vi "Test Host Image Acquisition Module Random Data No Accumulation.vi"(8 "error in":errorcluster, 11 "Operation":T3) -> (0 "error out":errorcluster, 1 "Image Acquired":bool, 2 "Acq In Progress":bool, 3 "Image":T2(plugin-control))   [LabVIEW 2013]
uses:
  Host/Image Acquisition/Host Image Acquisition Module Enum.ctl
  Host/Image Acquisition/Acquisition Settings Cluster.ctl
  <vilib>/vision/Image Controls.llb/IMAQ Image.ctl
  Host/Image Acquisition/Image Acquisition Settings FG Enum.ctl
  Host/System Status/Status FG Enum.ctl
  Host/Image Processing/Mask ROI FG Enum.ctl
  <vilib>/Utility/error.llb/Error Cluster From Error Code.vi
  <vilib>/rvi/errors/niLvFpgaAdjustHostInterfaceError.vi
  <vilib>/FPGAPlugInAG/PCIe-7842R/niLvFpga_Run_PCIe-7842R.vi
  <vilib>/FPGAPlugInAG/PCIe-7842R/niLvFpga_Close_PCIe-7842R.vi
  <vilib>/rvi/interface/nirviReadWriteControl/nirviReadWriteControl.xnode
  Host/FGs/FPGA_Reference.ctl
  Common/CL Configuration.ctl
  Common/CL Signal Mapping.ctl
  FPGA Bitfiles/WingBeatAnalyzer_FPGATargetSim_10_2.lvbitx
  <vilib>/rvi/interface/nirviMethod/nirviMethod.xnode
  FPGA/Sector/Accumulate/Sector Parameter Cluster.ctl
  <vilib>/rvi/interface/nirviCloseFPGA/nirviCloseFPGA.xnode
  Common/Timing/Timing Lib.lvlib
  Host/Globals/Average Sector Data.vi
  NiFpgaLv.dll
  <vilib>/FPGAPlugInAG/PCIe-7842R/niLvFpga_ConfigureFifo_PCIe-7842R.vi
  <vilib>/rvi/errors/niLvFpgaMergeErrorWithErrorCode.vi
  <vilib>/FPGAPlugInAG/PCIe-7842R/niLvFpga_StartFifo_PCIe-7842R.vi
  <vilib>/FPGAPlugInAG/PCIe-7842R/niLvFpga_ReadFifo_PCIe-7842R.vi
  <vilib>/FPGAPlugInAG/PCIe-7842R/niLvFpga_Reset_PCIe-7842R.vi
panel:
  out "Actual Depth":u32
  out "Target Sim TO":bool
  out "Cam Data Timeout":bool
  out "Sector FIFO Timeout":bool
  out "Host DMA Timeout":bool
  out "Number of Elements to Write Host DMA":u32
  out "Number of Elements to Read Cam Data":u32
  out "Image Data":u64[](array[numeric])
  out "Elements Remaining":u32
  out "Words per image":u32
  out "Num Frames read":u32
  out "DMA Words per Image":u32
  out "Acquire":bool
  in  "Acquisition Settings Cluster":T1={"Image Width"=2040, "Image Height"=1088, "Frames To Acquire"=0, "Signal Mapping"=enum."Basler 10-tap", "DMA Buffer Size\n(In Images)"=64} {"Image Height" max=65535; "Image Width" max=65535 step=40}
  out "Buffer Size":u32
  out "Acq'd Frame Width":u32=2040
  out "DMA Write Timeout":bool
  in  "Start Serial Server":bool
  out "Frames Acq'd":u32=1
  out "Acq'd Frame Height":u32=1088
  out "Initialized":bool
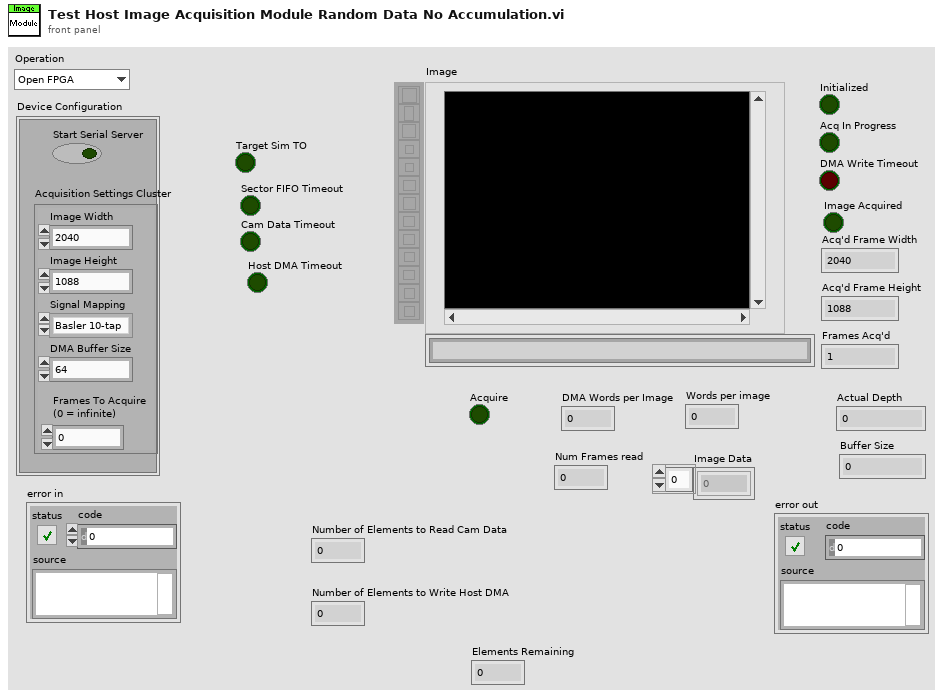
[diagram p1: front panel]
types:
  T1 = typedef "Acquisition Settings Cluster.ctl" = cluster{"Image Width":u32, "Image Height":u32, "Frames To Acquire":u32, "Signal Mapping":enum8{"Standard", "Basler 10-tap", "Vosskühler 10-tap"}, "DMA Buffer Size\n(In Images)":u32}
  T2 = typedef "IMAQ Image.ctl" = refnum<image>
  T3 = typedef "Host Image Acquisition Module Enum.ctl" = enum16{"Open FPGA", "Initialize DMA FIFO", "Load Sim Images", "Initialize Acquisition", "Update Sector Parameters", "Start Acquisition", "Aquire Image", "Read Averages", "Cancel Acquisition", "Close FPGA"}
  T4 = enum8{"Standard", "Basler 10-tap", "Vosskühler 10-tap"}
  T5 = typedef "Image Acquisition Settings FG Enum.ctl" = enum16{"Read", "Write"}
  T6 = typedef "Status FG Enum.ctl" = enum16{"Reset", "Read", "Write"}
  T7 = typedef "Mask ROI FG Enum.ctl" = enum16{"Read", "Write"}
  T8 = enum16{"big-endian, network order", "native, host order", "little-endian"}
  T9 = typedef "FPGA_Reference.ctl" = refnum<k20>
  T10 = typedef "Image Type" = u32
  T11 = typedef "Mask ROI Cluster.ctl" = cluster{"left annulus":T12, "right annulus":T12, "Threshold Range":cluster{"Lower value":dbl, "Upper value":dbl}, "[Avg BG]":u8[], "Number of Sectors":u8, "Left ROI":T13, "Right ROI":T13, "Left Start Angle Duty Cycle":fxp<+,8,0>, "Left End Angle Duty Cycle":fxp<+,8,0>, "Right End Angle Duty Cycle":fxp<+,8,0>, "Right Start Angle Duty Cycle":fxp<+,8,0>, "[Sector ROIs]":T13[]}
  T12 = typedef "IMAQ Circle" = cluster{"Center X":i32, "Center Y":i32, "Inner Radius":i32, "Outer Radius":i32, "Start Angle":dbl, "End Angle":dbl}
  T13 = typedef "ROI Descriptor" = cluster{"Global Rectangle":i32[], "Contours":cluster{"ID":enum32{"External", "Internal"}, "Type":u32, "Coordinates":i32[]}[]}
  T14 = typedef "Sector Parameter Cluster.ctl" = cluster{"Start Angle":fxp<+/-,17,2>, "End Angle":fxp<+,17,3>, "Inner Radius":u16, "Outter Radius":u16, "Hinge X":u16, "Hinge Y":u16, "NumWingSectors":u8}
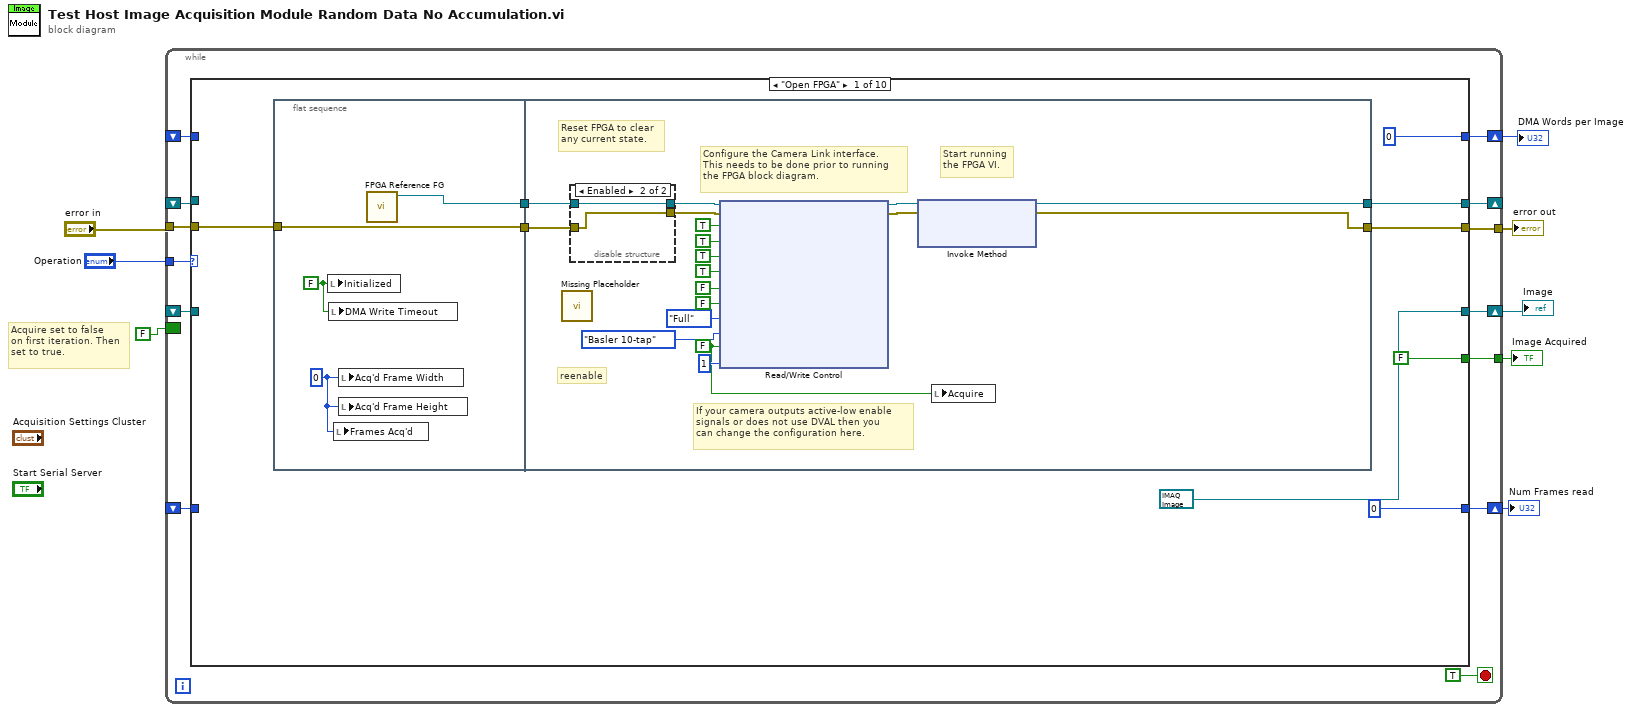
[diagram p0: block diagram]
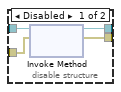
[diagram p2: hidden frame]
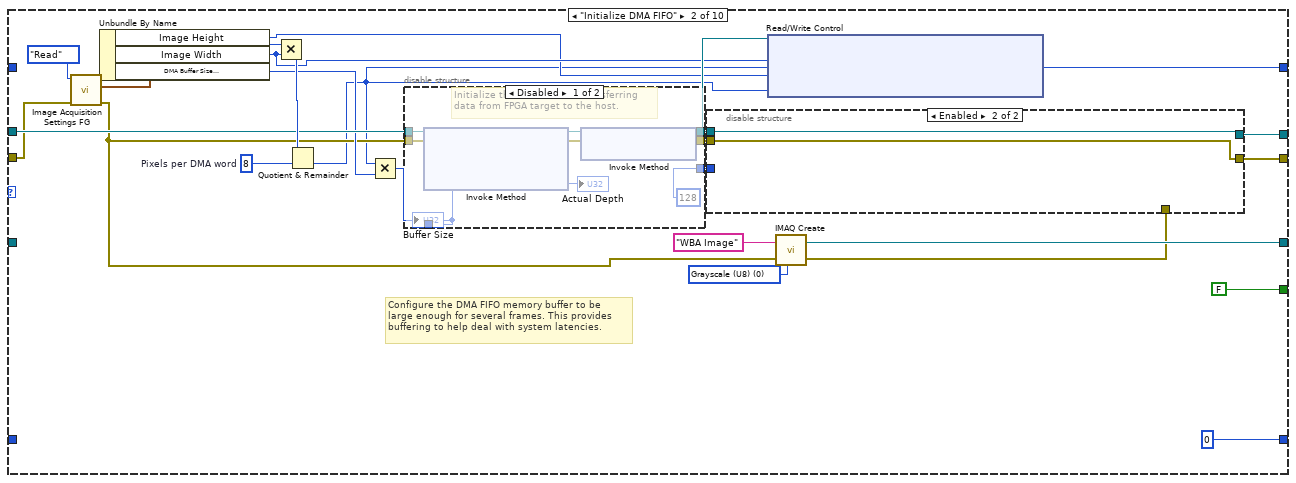
[diagram p3: hidden frame]
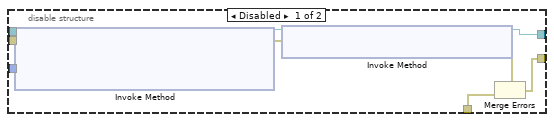
[diagram p5: hidden frame]
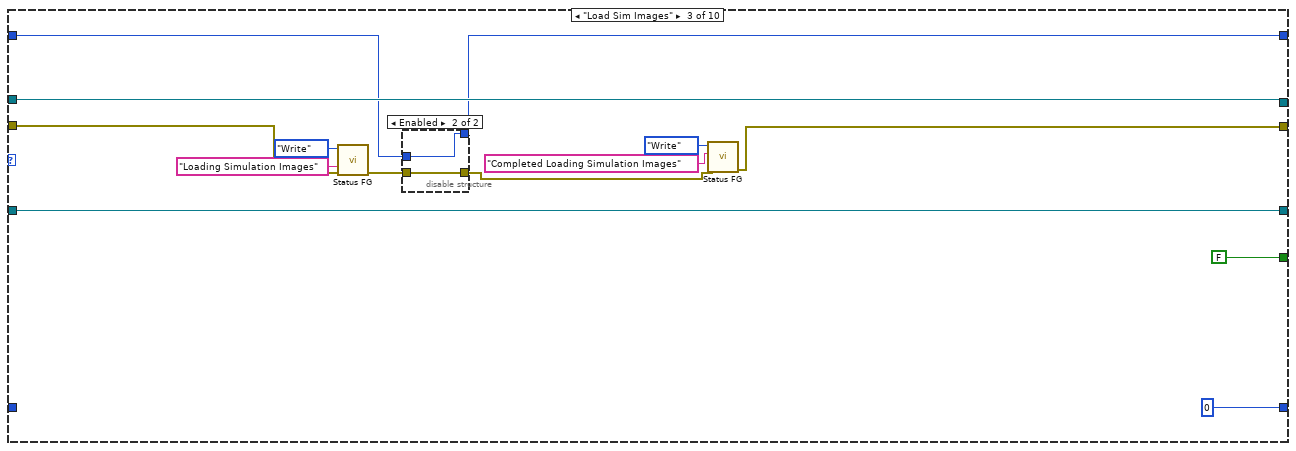
[diagram p6: hidden frame]
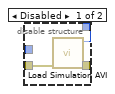
[diagram p7: hidden frame]
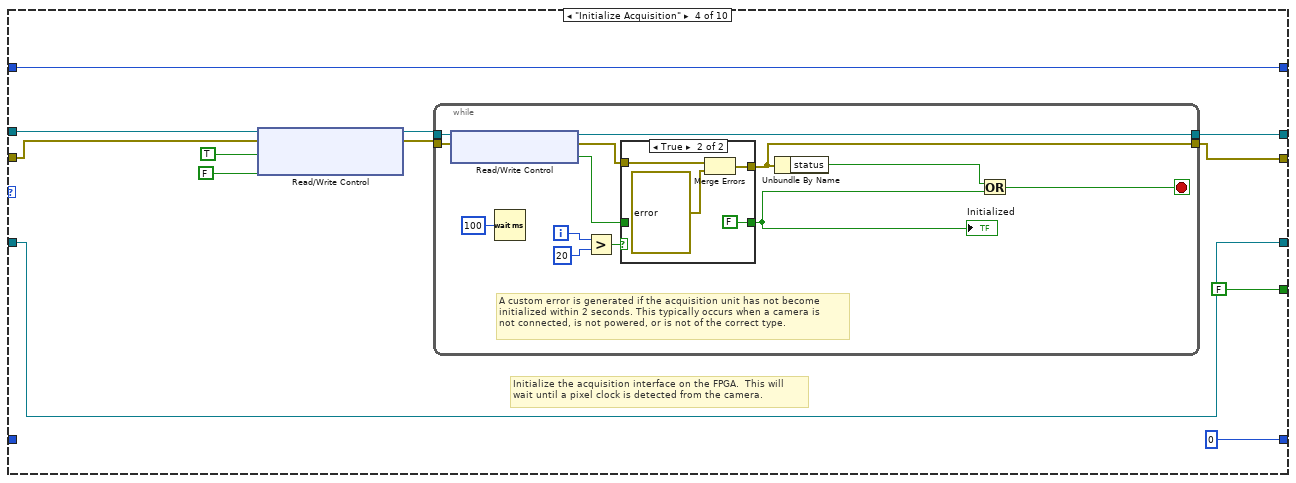
[diagram p8: hidden frame]
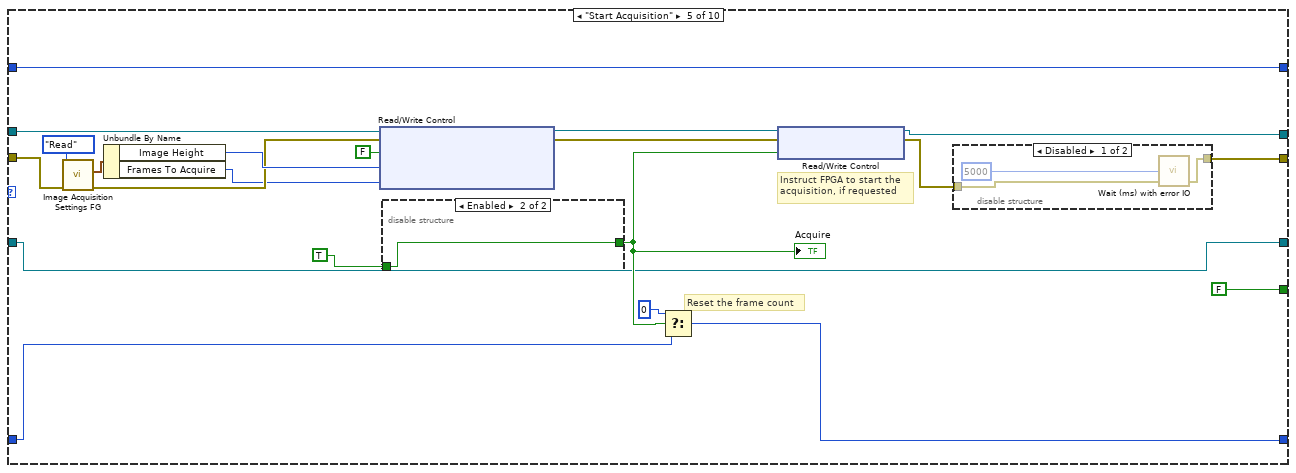
[diagram p10: hidden frame]
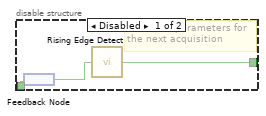
[diagram p12: hidden frame]
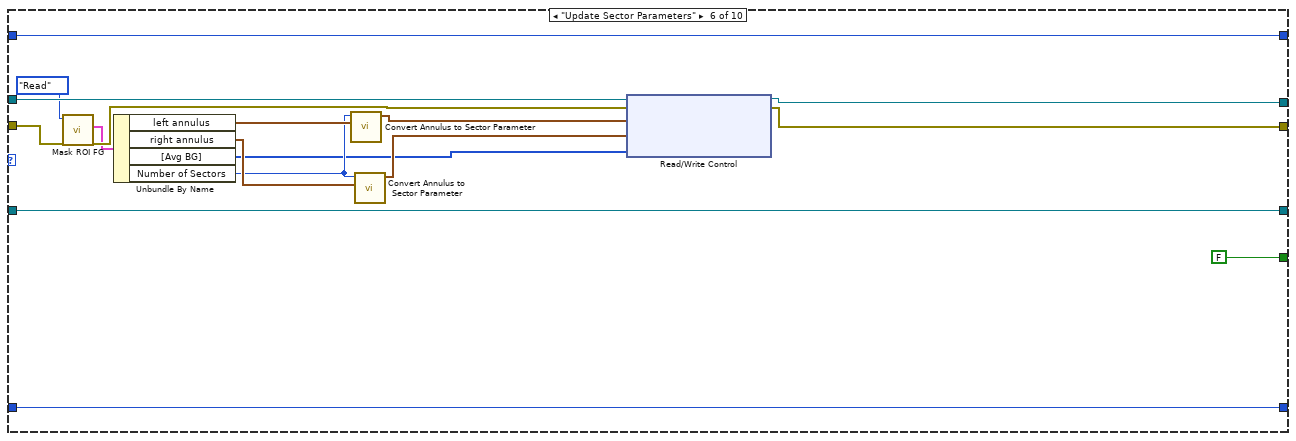
[diagram p13: hidden frame]
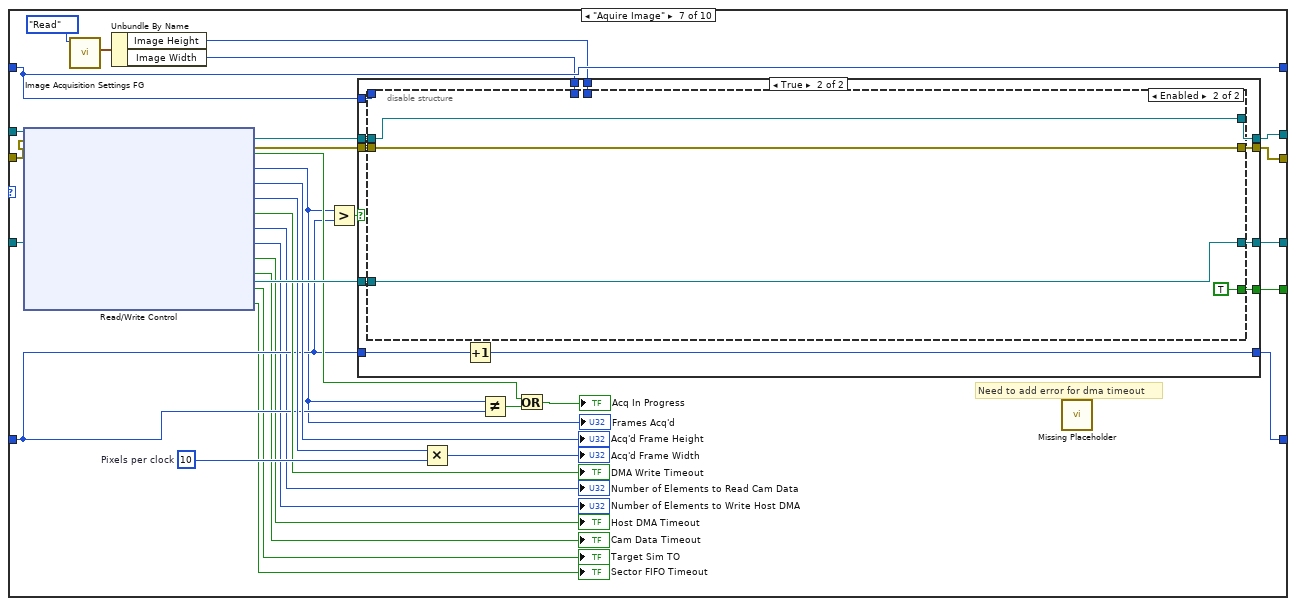
[diagram p14: hidden frame]
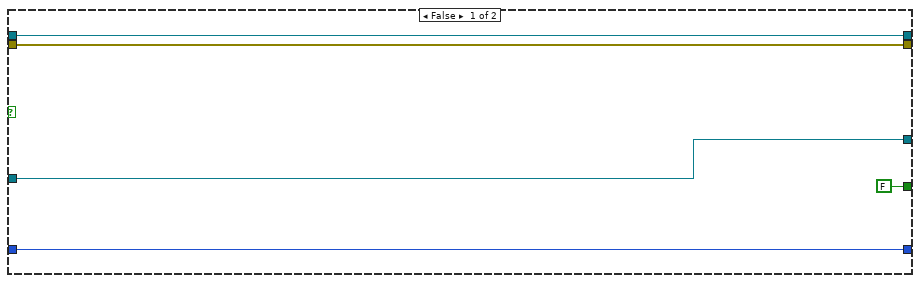
[diagram p15: hidden frame]
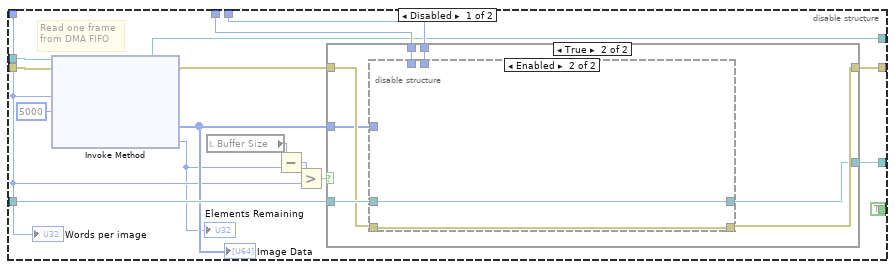
[diagram p16: hidden frame]
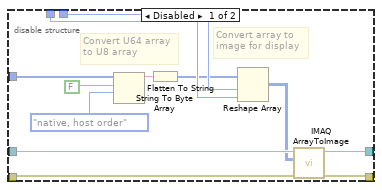
[diagram p18: hidden frame]
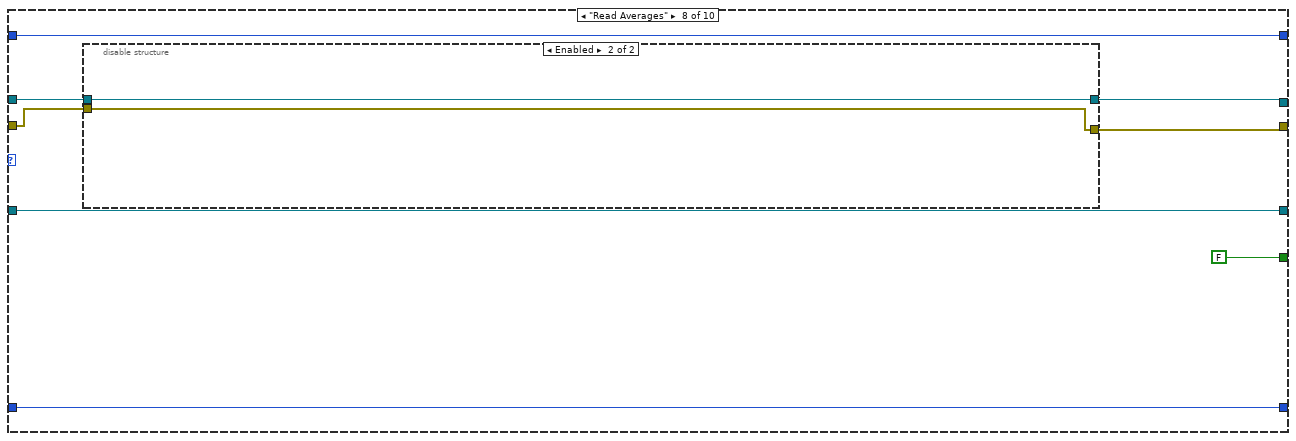
[diagram p19: hidden frame]
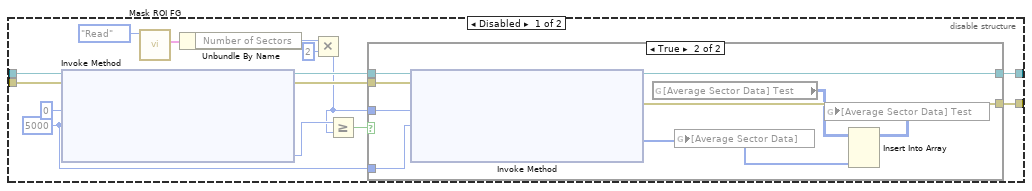
[diagram p20: hidden frame]
diagram:
  # "Acquire set to false\non first iteration. Then\nset to true."
  n1 = while {
    shift-right: [w20] -> _
    shift-left: _ -> [w16]
    tunnel: "error in" -> [w19]
    tunnel: "Operation" -> [w18]
    tunnel: [w17] -> w6
    shift-right: [w15] -> w3
    shift-left: _ -> [w14]
    shift-right: [w13] -> w4
    shift-left: _ -> [w10]
    shift-right: [w12] -> w2
    shift-left: _ -> [w11]
    border: FALSE ("Acquire") -> [_]
    tunnel: [w9] -> w1
    stop <- TRUE stop-if-true
    n2 = case shown="\"Open FPGA\"" w18 {
      tunnel: w19 -> [w30 w71 w112 w124 w167 w197 w212 w293 w333 w339]
      tunnel: [w29 w65 w115 w130 w160 w193 w230 w299 w335 w340] -> w20
      tunnel: [w28 w66 w106 w126 w158 w194 w229 w294 w332 w346] -> w17
      tunnel: w16 -> [_ w78 w115 w131 w168 w199 w231 w300 w337 w342]
      tunnel: [u32 0 w59 w114 w129 w163 w198 w222 w298 w331 w343] -> w15
      tunnel: w14 -> [_ _ w104 w129 w163 w198 w222 w298 w331 w343]
      tunnel: [T2 refnum ("New Image") w74 w116 w125 w162 w184 w224 w297 w334 w344] -> w13
      tunnel: [u32 0 u32 0 u32 0 u32 0 w164 w192 w228 w296 u32 0 w345] -> w12
      tunnel: w11 -> [_ _ _ _ w165 w192 w210 w296 _ w345]
      tunnel: w10 -> [_ _ w116 w125 w162 w184 w223 w297 w334 w344]
      tunnel: [FALSE ("Image Acquired") FALSE ("Image Acquired") FALSE ("Image Acquired") FALSE ("Image Acquired") FALSE ("Image Acquired") FALSE ("Image Acquired") w204 FALSE ("Image Acquired") FALSE ("Image Acquired") FALSE ("Image Acquired")] -> w9
      frame "Open FPGA" {
        n3 = flat-sequence {
          tunnel: w30 -> [w31]
          tunnel: [w32] -> w27
          tunnel: [w31] -> w26
          tunnel: [w37] -> w28
          tunnel: [w38] -> w29
          tunnel: w27 -> [w42]
          tunnel: w26 -> [w39]
          frame #0 {
            w33 = u32 0 ("Acq'd Frame Width")
            w34 = FALSE ("Initialized")
            n4 = local write "Initialized"(w34) -> ()
            n5 = local write "DMA Write Timeout"(w34) -> ()
            n6 = local write "Frames Acq'd"(w33) -> ()
            n7 = local write "Acq'd Frame Width"(w33) -> ()
            n8 = local write "Acq'd Frame Height"(w33) -> ()
            n9 = call "FPGA Reference FG.vi"() -> ("FPGA VI Reference Out"=w32:T9)  [unwired: 11 in]
          }
          frame #1 {
            w35 = FALSE ("Acq Control.Acquire")
            # "reenable"
            # "If your camera outputs active-low enable\nsignals or does not use DVAL then you \ncan change the configuration here."
            # "Start running\nthe FPGA VI."
            # "Reset FPGA to clear\nany current state."
            # "Configure the Camera Link interface.\nThis needs to be done prior to running\nthe FPGA block diagram."
            n10 = call "Missing Placeholder.vi"() -> ()  [unwired: 12 in]
            n11 = disable-structure shown="Enabled" {
              disable-tunnel: [w56 w58] -> w46
              disable-tunnel: [w55 w57] -> w44
              disable-tunnel: w42 -> [w54 w58]
              disable-tunnel: w39 -> [w53 w57]
              frame Disabled {
                n12 = xnode "Invoke Method"("FPGA VI Reference In"=w54, "error in"=w53) -> ("FPGA VI Reference Out"=w56:T9, "error out"=w55:errorcluster)
              }
              frame Enabled {
              }
            }
            n13 = xnode "Read/Write Control"("FPGA VI Reference In"=w46, "error in"=w44, "CL Config.FVAL Active High"=TRUE ("IO Module Config.CL FVAL Active High"), "CL Config.LVAL Active High"=TRUE ("IO Module Config.CL LVAL Active High"), "CL Config.DVAL Active High"=TRUE ("IO Module Config.CL DVAL Active High"), "CL Config.Spare Active High"=TRUE ("IO Module Config.CL Spare Active High"), "CL Config.Line Scan"=FALSE, "Acq Control.Ignore DVAL"=FALSE ("CL Config.Line Scan"), "CL Config.Configuration"=enum8{"Base", "Medium", "Full"}."Full", "CL Config.Signal Mapping"=T4."Basler 10-tap", "Acq Control.Acquire"=w35, "# of Frames to Average"=u8 1) -> ("FPGA VI Reference Out"=w43:T9, "error out"=w45:errorcluster)
            n14 = xnode "Invoke Method"("FPGA VI Reference In"=w43, "error in"=w45) -> ("FPGA VI Reference Out"=w38:T9, "error out"=w37:errorcluster)  [unwired: 1 in]
            n15 = local write "Acquire"(w35) -> ()
          }
        }
      }
      frame "Initialize DMA FIFO" {
        w75 = T10 0 items=["Grayscale (U8)", "Grayscale (I16)", "Grayscale (SGL)", "Complex (CSG)", "RGB (U32)", "HSL (U32)", "RGB (U64)", "Grayscale (U16)"] ("Image Type")
        w80 = u32 8  # Pixels per DMA word
        # "Configure the DMA FIFO memory buffer to be\nlarge enough for several frames. This provides\nbuffering to help deal with system latencies."
        n16 = call "Image Acquisition Settings FG.vi"("error in (no error)"=w71, "Operation"=Image_Acquisition_Settings_FG_Enum."Read") -> ("error out"=w68:errorcluster, "Acquisition Settings Out"=w72:T1)  [unwired: 8 in]
        n17 = Unbundle By Name(w72) -> ("Image Height"=w60:u32, "Image Width"=w61:u32, "DMA Buffer Size\n(In Images)"=w70:u32)
        n18 = Multiply(x=w60, y=w61) -> (x*y=w79:u32)
        n19 = Quotient & Remainder(x=w79, y=w80) -> (floor(x/y)=w59:u32)  [unwired: 1 out]
        n20 = Multiply(x=w59, y=w70) -> (x*y=w81:u32)
        n21 = disable-structure shown="Disabled" {
          disable-tunnel: w81 -> [w90 _]
          disable-tunnel: w78 -> [w89 w92]
          disable-tunnel: [u32 128 ("Requested Depth") _] -> w69
          disable-tunnel: w68 -> [w87 w91]
          disable-tunnel: [w86 w91] -> w63
          disable-tunnel: [w85 w92] -> w62
          frame Disabled {
            # "Initialize the DMA FIFO for transferring\ndata from FPGA target to the host."
            n22 = xnode "Invoke Method"("FPGA VI Reference In"=w89, "error in"=w87, "Requested Depth"=w90) -> ("FPGA VI Reference Out"=w84:T9, "error out"=w83:errorcluster, "Actual Depth"=→"Actual Depth":u32)
            n23 = xnode "Invoke Method"("FPGA VI Reference In"=w84, "error in"=w83) -> ("FPGA VI Reference Out"=w85:T9, "error out"=w86:errorcluster)
            "Buffer Size" <- w90
          }
          frame Enabled {
          }
        }
        n24 = xnode "Read/Write Control"("FPGA VI Reference In"=w62, "X Resolution"=w61, "Y Resolution"=w60, "Words per image"=w59) -> ()  [unwired: 1 in, 2 out]
        n25 = call "IMAQ Create"("Image Name"="WBA Image", "Image Type"=w75, "error in (no error)"=w68) -> ("New Image"=w74:T2, "error out"=w67:errorcluster)  [unwired: 2 in]
        n26 = disable-structure shown="Enabled" {
          disable-tunnel: w69 -> [w101 _]
          disable-tunnel: w67 -> [w98 _]
          disable-tunnel: [w96 w102] -> w66
          disable-tunnel: [w95 w103] -> w65
          disable-tunnel: w62 -> [w94 w103]
          disable-tunnel: w63 -> [w93 w102]
          frame Disabled {
            n27 = xnode "Invoke Method"("FPGA VI Reference In"=w94, "error in"=w93, "Requested Depth"=w101) -> ("FPGA VI Reference Out"=w100:T9, "error out"=w99:errorcluster)  [unwired: 1 out]
            n28 = xnode "Invoke Method"("FPGA VI Reference In"=w100, "error in"=w99) -> ("FPGA VI Reference Out"=w95:T9, "error out"=w97:errorcluster)
            n29 = Merge Errors(w97, w98) -> (w96:errorcluster)
          }
          frame Enabled {
          }
        }
      }
      frame "Load Sim Images" {
        n30 = call "Status FG.vi"("error in (no error)"=w112, "Status In"="Loading Simulation Images", "Operation"=Status_FG_Enum."Write") -> ("error out"=w111:errorcluster)  [unwired: 7 in, 1 out]
        n31 = disable-structure shown="Enabled" {
          disable-tunnel: [w120 w121] -> w114
          disable-tunnel: w111 -> [w119 w122]
          disable-tunnel: [w118 w122] -> w107
          disable-tunnel: w104 -> [_ w121]
          frame Disabled {
            n32 = call "Load Simulation AVI.vi"("error in (no error)"=w119) -> ("error out"=w118:errorcluster, "Words per image"=w120:u32)  [unwired: 9 in]
          }
          frame Enabled {
          }
        }
        n33 = call "Status FG.vi"("error in (no error)"=w107, "Status In"="Completed Loading Simulation Images", "Operation"=Status_FG_Enum."Write") -> ("error out"=w106:errorcluster)  [unwired: 7 in, 1 out]
      }
      frame "Initialize Acquisition" {
        # "Initialize the acquisition interface on the FPGA.  This will\nwait until a pixel clock is detected from the camera."
        n34 = xnode "Read/Write Control"("FPGA VI Reference In"=w131, "error in"=w124, "Acq Control.Initialize"=TRUE ("Arm Acquisition"), "Acq Control.Cancel Acq"=FALSE) -> ("FPGA VI Reference Out"=w134:T9, "error out"=w133:errorcluster)
        n35 = while {
          tunnel: w134 -> [w143]
          tunnel: w133 -> [w142]
          tunnel: [w141] -> w130
          tunnel: [w144] -> w126
          i -> [w137]
          stop <- w147 stop-if-true
          # "A custom error is generated if the acquisition unit has not become\ninitialized within 2 seconds. This typically occurs when a camera is\nnot connected, is not powered, or is not of the correct type."
          n36 = xnode "Read/Write Control"("FPGA VI Reference In"=w143, "error in"=w142) -> ("FPGA VI Reference Out"=w141:T9, "error out"=w140:errorcluster, "Acq Status.Initialized"=w139:bool)
          n37 = Wait (ms)(milliseconds to wait=u32 100) -> ()  [unwired: 1 out]
          n38 = Greater?(x=w137, y=20) -> (0:w138:bool)
          n39 = case shown="True" w138 {
            tunnel: [w149 FALSE] -> w135
            tunnel: w139 -> [w149 _]
            tunnel: w140 -> [w148 w151]
            tunnel: [w148 w153] -> w144
            frame False {
            }
            frame True {
              n40 = Merge Errors(w151, errorcluster {"status"=TRUE, "code"=-8999, "source"="Acquisition Initialization: This error typically occurs when a camera is not properly connected, is not powered, or is not of the correct type."} ("error in")) -> (w153:errorcluster)
            }
          }
          "Initialized" <- w135
          n41 = Unbundle By Name(w144) -> ("status"=w146:bool)
          n42 = Or(x=w146, y=w135) -> (x .or. y?=w147:bool)
        }
      }
      frame "Start Acquisition" {
        # "Reset the frame count"
        # "Instruct FPGA to start the\nacquisition, if requested"
        n43 = call "Image Acquisition Settings FG.vi"("error in (no error)"=w167, "Operation"=Image_Acquisition_Settings_FG_Enum."Read") -> ("error out"=w166:errorcluster, "Acquisition Settings Out"=w174:T1)  [unwired: 8 in]
        n44 = Unbundle By Name(w174) -> ("Image Height"=w169:u32, "Frames To Acquire"=w156:u32)
        n45 = xnode "Read/Write Control"("FPGA VI Reference In"=w168, "error in"=w166, "Acq Control.Cancel Acq"=FALSE, "Acq Control.Line Scan Height"=w169, "Acq Control.Frames To Acq"=w156) -> ("FPGA VI Reference Out"=w154:T9, "error out"=w155:errorcluster)
        n46 = disable-structure shown="Enabled" {
          disable-tunnel: [w181 w182] -> w171
          disable-tunnel: TRUE ("Acquire") -> [w179 w182]
          frame Disabled {
            # "Write the parameters for\nthe next acquisition"
            n47 = feedback #1() -> (w180:bool)
            n48 = feedback-in #1(w179) -> ()
            n49 = call "Rising Edge Detect.vi"("Input"=w180) -> ("Pulse"=w181:bool)  [unwired: 4 in]
          }
          frame Enabled {
          }
        }
        "Acquire" <- w171
        n50 = Select(t=u32 0, s=w171, f=w165) -> (s? t:f=w164:u32)
        n51 = xnode "Read/Write Control"("FPGA VI Reference In"=w154, "error in"=w155, "Acq Control.Acquire"=w171) -> ("FPGA VI Reference Out"=w160:T9, "error out"=w159:errorcluster)
        n52 = disable-structure shown="Disabled" {
          disable-tunnel: w159 -> [w176 w178]
          disable-tunnel: [w175 w178] -> w158
          frame Disabled {
            n53 = call "Wait (ms) with error IO.vi"("error in (no error)"=w176, "milliseconds to wait"=u32 5000) -> ("error out"=w175:errorcluster)  [unwired: 3 in]
          }
          frame Enabled {
          }
        }
      }
      frame "Update Sector Parameters" {
        n54 = call "Mask ROI FG.vi"("error in (no error)"=w197, "Operation"=Mask_ROI_FG_Enum."Read") -> ("error out"=w196:errorcluster, "Mask ROI Out"=w191:T11)  [unwired: 8 in]
        n55 = Unbundle By Name(w191) -> ("left annulus"=w190:T12, "right annulus"=w188:T12, "[Avg BG]"=w185:u8[], "Number of Sectors"=w187:u8)
        n56 = call "Convert Annulus to Sector Parameter.vi"("Annulus"=w190, "NumWingSectors"=w187) -> ("Sector Parameter"=w189:T14)  [unwired: 9 in]
        n57 = call "Convert Annulus to Sector Parameter.vi"("Annulus"=w188, "NumWingSectors"=w187) -> ("Sector Parameter"=w186:T14)  [unwired: 9 in]
        n58 = xnode "Read/Write Control"("FPGA VI Reference In"=w199, "error in"=w196, "Sector Parameters Left"=w189, "Sector Parameters Right"=w186, "[Average BG Intensity]"=w185) -> ("FPGA VI Reference Out"=w193:T9, "error out"=w194:errorcluster)
      }
      frame "Aquire Image" {
        w220 = u32 10  # Pixels per clock
        # "Need to add error for dma timeout"
        n59 = xnode "Read/Write Control"("FPGA VI Reference In"=w231, "error in"=w212) -> ("FPGA VI Reference Out"=w227:T9, "error out"=w226:errorcluster, "Acq Status.Acq In Progress"=w211:bool, "Acq Status.Frames Acq'd"=w209:u32, "Acq Status.Lines Per Frame"=→"Acq'd Frame Height":u32, "Acq Status.Clocks Per Line"=w219:u32, "Acq Status.DMA Write Timeout"=→"DMA Write Timeout":bool, "Number of Elements to Read Cam Data"=→"Number of Elements to Read Cam Data":u32, "Number of Elements to Write Host DMA"=→"Number of Elements to Write Host DMA":u32, "Host DMA Timeout"=→"Host DMA Timeout":bool, "Cam Data Timeout"=→"Cam Data Timeout":bool, "Target Sim TO"=→"Target Sim TO":bool, "Sector FIFO Timeout"=→"Sector FIFO Timeout":bool)
        "Frames Acq'd" <- w209
        n60 = call "Image Acquisition Settings FG.vi"("Operation"=Image_Acquisition_Settings_FG_Enum."Read") -> ("Acquisition Settings Out"=w215:T1)  [unwired: 9 in, 1 out]
        n61 = Unbundle By Name(w215) -> ("Image Height"=w214:u32, "Image Width"=w213:u32)
        n62 = Greater?(x=w209, y=w210) -> (0:w225:bool)
        n63 = case shown="True" w225 {
          tunnel: w227 -> [w235 w238]
          tunnel: w226 -> [w234 w239]
          tunnel: w214 -> [_ w248]
          tunnel: w213 -> [_ w247]
          tunnel: w223 -> [w236 w246]
          tunnel: [w234 w245] -> w229
          tunnel: [w235 w244] -> w230
          tunnel: w210 -> [w233 w243]
          tunnel: [w233 w242] -> w228
          tunnel: w222 -> [_ w241]
          tunnel: [w236 w240] -> w224
          tunnel: [FALSE ("Image Acquired") w237] -> w204
          frame False {
          }
          frame True {
            n64 = disable-structure shown="Enabled" {
              disable-tunnel: w248 -> [w265 _]
              disable-tunnel: w247 -> [w264 _]
              disable-tunnel: w246 -> [w263 w289]
              disable-tunnel: [w261 w291] -> w245
              disable-tunnel: [w260 w290] -> w244
              disable-tunnel: w241 -> [w257 _]
              disable-tunnel: [w256 w289] -> w240
              disable-tunnel: w239 -> [w251 w291]
              disable-tunnel: w238 -> [w250 w290]
              disable-tunnel: [TRUE ("Image Acquired") TRUE ("Image Acquired")] -> w237
              frame Disabled {
                # "Read one frame\nfrom DMA FIFO"
                n65 = xnode "Invoke Method"("FPGA VI Reference In"=w250, "error in"=w251, "Number of Elements"=w257, "Timeout (ms)"=5000) -> ("FPGA VI Reference Out"=w260:T9, "error out"=w262:errorcluster, "Data"=w259:u64[], "Elements Remaining"=w254:u32)
                "Elements Remaining" <- w254
                "Image Data" <- w259
                n66 = local read "Buffer Size"() -> (w255:u32)
                n67 = Subtract(x=w255, y=w254) -> (x-y=w253:u32)
                n68 = Greater?(x=w253, y=w257) -> (0:w258:bool)
                n69 = case shown="True" w258 {
                  tunnel: w265 -> [_ w274]
                  tunnel: w264 -> [_ w273]
                  tunnel: w263 -> [w266 w272]
                  tunnel: w262 -> [w267 w271]
                  tunnel: [w267 w270] -> w261
                  tunnel: w259 -> [_ w269]
                  tunnel: [w266 w268] -> w256
                  frame False {
                    # "Do not display the image if we're\nfalling behind in the acquisition."
                  }
                  frame True {
                    n70 = disable-structure shown="Enabled" {
                      disable-tunnel: w274 -> [w286 _]
                      disable-tunnel: w273 -> [w285 _]
                      disable-tunnel: w272 -> [w284 w288]
                      disable-tunnel: w271 -> [w283 w287]
                      disable-tunnel: [w282 w287] -> w270
                      disable-tunnel: w269 -> [w279 _]
                      disable-tunnel: [w275 w288] -> w268
                      frame Disabled {
                        # "Convert U64 array\nto U8 array"
                        # "Convert array to\nimage for display"
                        n71 = Flatten To String(anything=w279, prepend array or string size? (T)=FALSE, byte order (0:big-endian, network order)=T8."native, host order") -> (data string=w277:string)  [unwired: 1 in, 2 out]
                        n72 = String To Byte Array(string=w277) -> (unsigned byte array=w276:u8[])
                        n73 = Reshape Array(w276, w286, w285) -> (w281:u8[][])
                        n74 = call "IMAQ ArrayToImage"("error in (no error)"=w283, "Image Pixels (U8)"=w281, "Image"=w284) -> ("error out"=w282:errorcluster, "Image Out"=w275:T2)  [unwired: 7 in]
                      }
                      frame Enabled {
                      }
                    }
                  }
                }
                "Words per image" <- w257
              }
              frame Enabled {
              }
            }
            n75 = Increment(x=w243) -> (x+1=w242:u32)
          }
        }
        n76 = Multiply(x=w219, y=w220) -> (x*y=→"Acq'd Frame Width":u32)
        n77 = Not Equal?(x=w209, y=w210) -> (x != y?=w208:bool)
        n78 = Or(x=w211, y=w208) -> (x .or. y?=→"Acq In Progress":bool)
        n79 = call "Missing Placeholder.vi"() -> ()  [unwired: 12 in]
      }
      frame "Read Averages" {
        n80 = disable-structure shown="Enabled" {
          disable-tunnel: w300 -> [w315 w328]
          disable-tunnel: [w310 w328] -> w299
          disable-tunnel: [w309 w327] -> w294
          disable-tunnel: w293 -> [w307 w327]
          frame Disabled {
            w311 = 5000 ("Timeout (ms)")
            n81 = xnode "Invoke Method"("FPGA VI Reference In"=w315, "error in"=w307, "Number of Elements"=u32 0, "Timeout (ms)"=w311) -> ("FPGA VI Reference Out"=w313:T9, "error out"=w312:errorcluster, "Elements Remaining"=w303:u32)  [unwired: 1 out]
            n82 = call "Mask ROI FG.vi"("Operation"=Mask_ROI_FG_Enum."Read") -> ("Mask ROI Out"=w306:T11)  [unwired: 9 in, 1 out]
            n83 = Unbundle By Name(w306) -> ("Number of Sectors"=w304:u8)
            n84 = Multiply(x=w304, y=u8 2) -> (x*y=w302:u8)
            n85 = Greater Or Equal?(x=w303, y=w302) -> (x >= y?=w305:bool)
            n86 = case shown="True" w305 {
              tunnel: w313 -> [w317 w326]
              tunnel: w312 -> [w316 w325]
              tunnel: w311 -> [_ w324]
              tunnel: [w317 w323] -> w310
              tunnel: [w316 w322] -> w309
              tunnel: w302 -> [_ w321]
              frame False {
              }
              frame True {
                n87 = xnode "Invoke Method"("FPGA VI Reference In"=w326, "error in"=w325, "Number of Elements"=w321, "Timeout (ms)"=w324) -> ("FPGA VI Reference Out"=w323:T9, "error out"=w322:errorcluster, "Data"=w319:u8[])  [unwired: 1 out]
                n88 = global read "Average Sector Data.vi" "[Average Sector Data] Test"() -> (w320:u8[][])
                n89 = global write "Average Sector Data.vi" "[Average Sector Data]"(w319) -> ()
                n90 = Insert Into Array(array=w320, new element=w319) -> (w318:u8[][])  [unwired: 2 in]
                n91 = global write "Average Sector Data.vi" "[Average Sector Data] Test"(w318) -> ()
              }
            }
          }
          frame Enabled {
          }
        }
      }
      frame "Cancel Acquisition" {
        n92 = xnode "Read/Write Control"("FPGA VI Reference In"=w337, "error in"=w333, "Acq Control.Cancel Acq"=TRUE) -> ("FPGA VI Reference Out"=w335:T9, "error out"=w332:errorcluster)
      }
      frame "Close FPGA" {
        n93 = xnode "Read/Write Control"("FPGA VI Reference In"=w342, "Acq Control.Cancel Acq"=TRUE) -> ("FPGA VI Reference Out"=w340:T9)  [unwired: 1 in, 1 out]
        n94 = xnode "Close FPGA VI Reference"("FPGA VI Reference In"=w340, "error in"=w339) -> ("error out"=w349:errorcluster)
        n95 = call <vilib>:"Simple Error Handler.vi"("error in (no error)"=w349) -> ("error out"=w347:errorcluster)  [unwired: 4 in, 4 out]
        n96 = call "IMAQ Dispose"("Image"=w344, "error in (no error)"=w347) -> ("error out"=w346:errorcluster)  [unwired: 4 in]
        n97 = local write "Initialized"(FALSE ("Initialized")) -> ()
      }
    }
  }
  "error out" <- w6
  "Image" <- w4
  "DMA Words per Image" <- w3
  "Num Frames read" <- w2
  "Image Acquired" <- w1
